vi "Send Save Process to Library.vi"(7 "Message Priority (Normal)":T1=enum."Normal", 8 "error in (no error)":errorcluster, 9 "Process":string, 10 "Library Path":path, 11 "Message Enqueuer":refnum<class "Message Enqueuer.lvclass">) -> (0 "error out":errorcluster, 3 "Message Enqueuer out":refnum<class "Message Enqueuer.lvclass">)   [LabVIEW 2016, in "CS++DSCManager.lvlib" / "Save Process to Library Msg.lvclass"]
doc: "Sends the <B>CS++DSCManager.lvlib:Save Process to Library Msg.lvclass</B> message.\n\n<B>CS++DSCManager.lvlib:CS++DSCManager.lvclass:Save Process to Library.vi</B> Description:\n\nSaves the deployed configuration of processes or shared variables to one or several LabVIEW project libraries."
uses:
  Save Process to Library Msg.lvclass
  <vilib>/ActorFramework/Message Enqueuer/Message Enqueuer.lvclass
  <vilib>/ActorFramework/Message Enqueuer/Message Priority.ctl
  C:/Program Files (x86)/National Instruments/LabVIEW 2016/vi.lib/ActorFramework/Message/Message.lvclass
  Save Process to Library Msg.lvclass/Save Process to Library Msg.ctl
  <vilib>/ActorFramework/Message Enqueuer/Message Enqueuer.lvclass/Message Enqueuer.ctl
  <vilib>/ActorFramework/Message Priority Queue/Priority Enqueue.vi
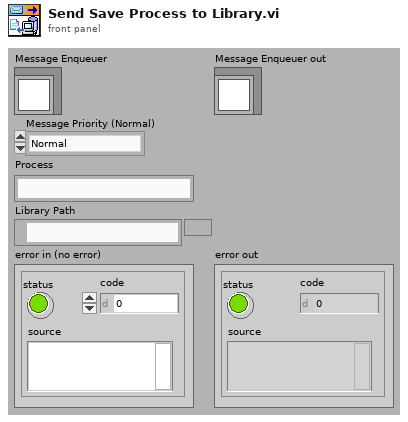
[diagram p1: front panel]
types:
  T1 = typedef "Actor Framework.lvlib/Message Enqueuer.lvclass/Message Priority.ctl" = enum16{"Low", "Normal", "High"}
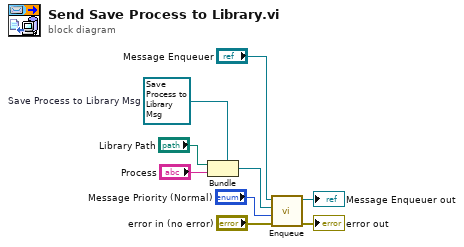
[diagram p0: block diagram]
diagram:
  w3 = refnum<class "Save Process to Library Msg.lvclass"> refnum  # Save Process to Library Msg
  n1 = Bundle(cluster=w3, "Library Path", "Process") -> (w6:refnum<class "Save Process to Library Msg.lvclass">)
  n2 = call <vilib>:"Enqueue.vi"("error in (no error)"="error in (no error)", "Message Priority (Normal)"="Message Priority (Normal)", "Message"=w6, "Message Enqueuer in"="Message Enqueuer") -> ("error out"=→"error out":errorcluster, "Message Enqueuer out"=→"Message Enqueuer out":refnum<class "Message Enqueuer.lvclass">)  [unwired: 6 in]
